vi "Launch Simulated Cars.vi"() -> ()   [LabVIEW 2017]
panel:
  in  "Destroy Sim Cars":bool
  in  "Generate Sim Cars":bool
  in  "# Cars":i32=1 min=1 max=20
  # "Simulated Car Launcher"
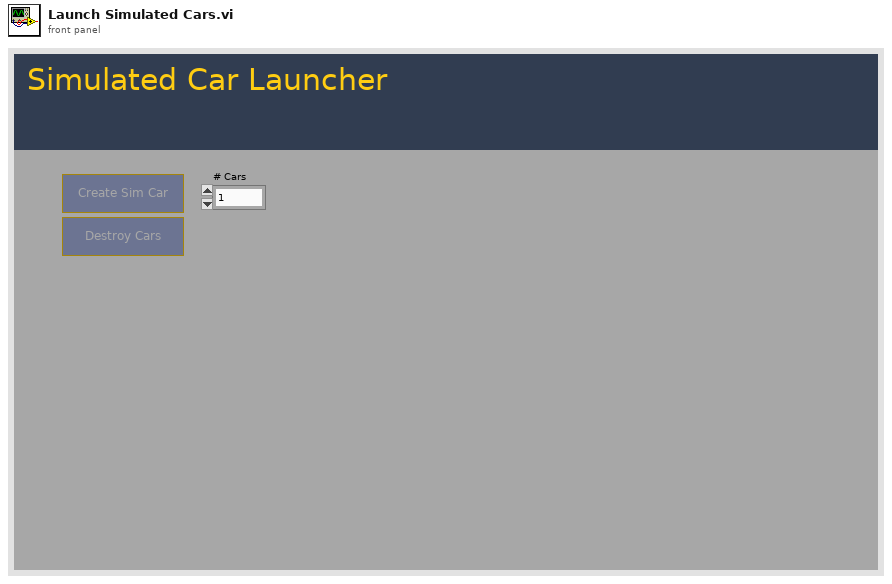
[diagram p1: front panel]
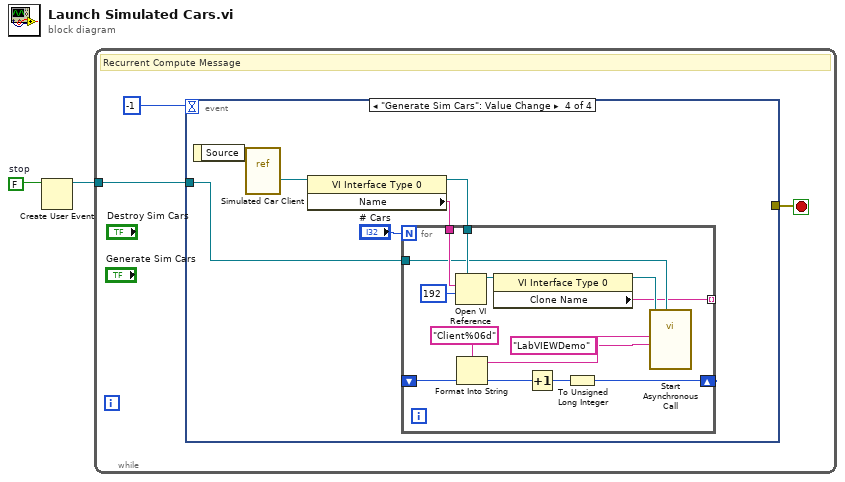
[diagram p0: block diagram]
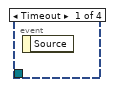
[diagram p2: hidden frame]
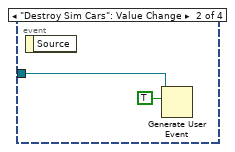
[diagram p3: hidden frame]
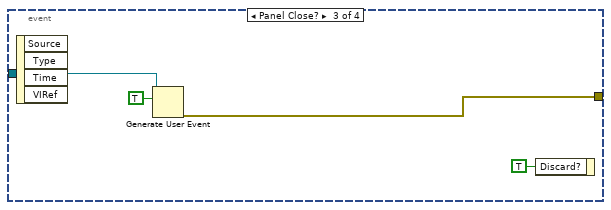
[diagram p4: hidden frame]
diagram:
  w2 = FALSE  # stop
  n1 = Create User Event(user event datatype=w2) -> (user event=w1:refnum<user-event>)  [unwired: 1 in, 1 out]
  n2 = while {
    tunnel: w1 -> [w5]
    stop <- w4 stop-if-true
    # "Recurrent Compute Message"
    n3 = event shown="[3] \"Generate Sim Cars\": Value Change" {
      selector: _ -> [_ _ _ _]
      dyn-events: _ -> [_ _ _ _]
      timeout: -1 -> [_ _ _ _]
      tunnel: w5 -> [_ w6 w10 w12]
      tunnel: [_ _ w9 _] -> w4
      event Timeout {
        n4 = event-data() -> ()  [unwired: 1 in, 1 out]
      }
      event "Destroy Sim Cars": Value Change {
        n5 = event-data() -> ()  [unwired: 1 in, 1 out]
        n6 = Generate User Event(user event=w6, event data cluster=TRUE ("event data")) -> ()  [unwired: 2 in, 2 out]
      }
      event Panel Close? {
        n7 = event-data() -> ()  [unwired: 1 in, 4 out]
        n8 = Generate User Event(user event=w10, event data cluster=TRUE ("event data")) -> (error out=w9:errorcluster)  [unwired: 2 in, 1 out]
        n9 = event-data("Discard?"=TRUE) -> ()  [unwired: 1 in, 1 out]
      }
      event "Generate Sim Cars": Value Change {
        n10 = event-data() -> ()  [unwired: 1 in, 1 out]
        n11 = vi-ref "Simulated Car Client.vi"() -> (w15:refnum<vi>)
        n12 = property class="VI Interface Type 0"(reference=w15) -> (reference out=w13:refnum<vi>, "Name"=w14:string)  [unwired: 1 in, 1 out]
        n13 = for {
          N: "# Cars" -> [_]
          tunnel: w14 -> [w28]
          tunnel: w13 -> [w27]
          tunnel: w12 -> [w26]
          shift-right: [w21] -> _
          shift-left: _ -> [w23]
          tunnel: [w18] -> _ mode=indexing
          n14 = Open VI Reference(type specifier VI Refnum (for type only)=w27, vi path=w28, options=192) -> (vi reference=w20:refnum<vi>)  [unwired: 3 in, 1 out]
          n15 = Format Into String(format string="Client%06d", w23) -> (resulting string=w25:string)  [unwired: 2 in, 1 out]
          n16 = property class="VI Interface Type 0"(reference=w20) -> (reference out=w19:refnum<vi>, "Clone Name"=w18:string)  [unwired: 1 in, 1 out]
          n17 = Increment(x=w23) -> (x+1=w22:u32)
          n18 = To Unsigned Long Integer(number=w22) -> (unsigned 32bit integer=w21:u32)
          n19 = call-by-ref "Start Asynchronous Call"(reference=w19, "stop signal"=w26, "project namespace"="LabVIEWDemo" ("format string"), "Client Name"=w25) -> ()  [unwired: 10 in, 2 out]
        }
      }
    }
  }
